vi "UtilityProcessCSVStringTo2DArray.vi"(8 "error in (no error)":errorcluster, 11 "CSV String":string) -> (0 "error out":errorcluster, 3 "Array":string[][](array[string]))   [LabVIEW 2019, in "flashcards.lvlib"]
uses:
  flashcards.lvlib
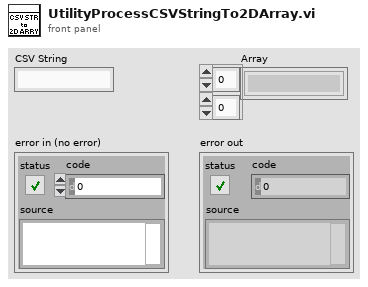
[diagram p1: front panel]
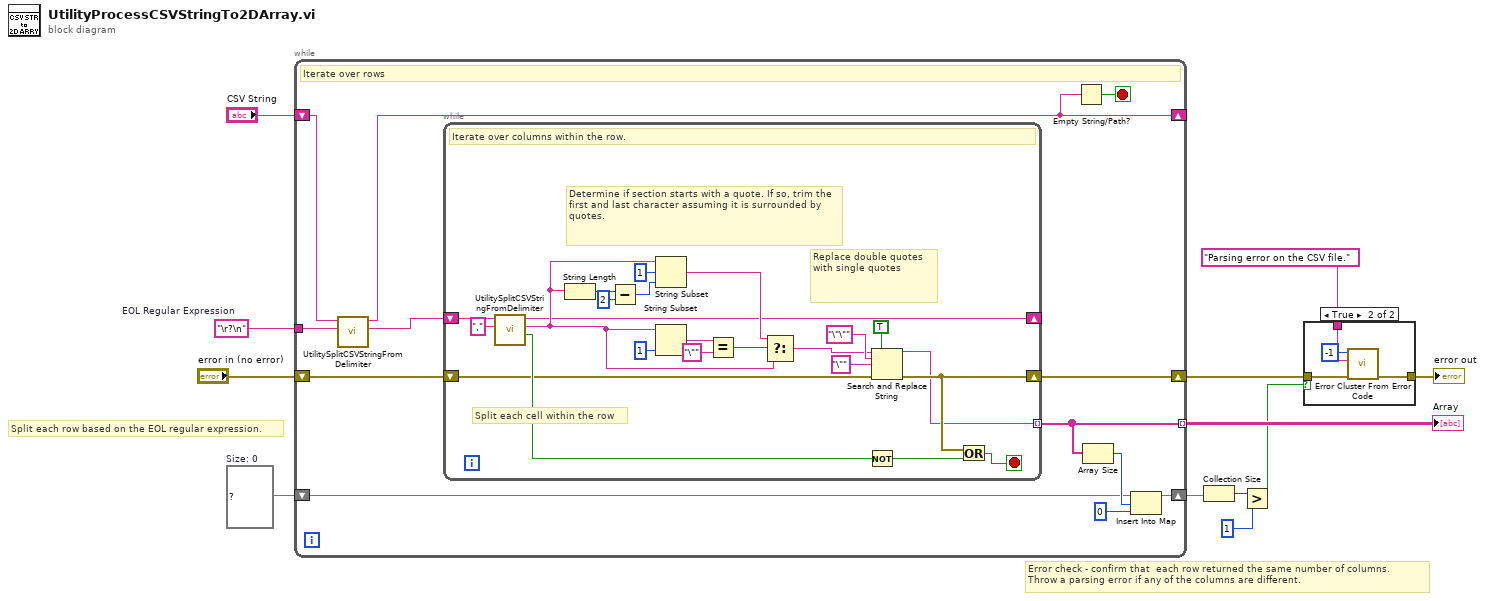
[diagram p0: block diagram]
diagram:
  w8 = map{i32, i32} {}  # Size: 0
  w12 = "\r?\n"  # EOL Regular Expression
  # "Error check - confirm that  each row returned the same number of columns.\nThrow a parsing error if any of the columns are different."
  # "Split each row based on the EOL regular expression."
  n1 = while {
    tunnel: w12 -> [w21]
    shift-right: [w23] -> w3
    shift-left: "error in (no error)" -> [w24]
    shift-right: [w20] -> _
    shift-left: "CSV String" -> [w19]
    tunnel: [w17] -> w11 mode=indexing
    shift-right: [w14] -> w7
    shift-left: w8 -> [w15]
    stop <- w22 stop-if-true
    # "Iterate over rows"
    n2 = call "UtilitySplitCSVStringFromDelimiter.vi"("Delimiter Regular Expression"=w21, "String in"=w19) -> ("Before Split"=w18:string, "After Split"=w20:string)  [unwired: 7 in, 1 out]
    n3 = while {
      shift-right: [w34] -> _
      shift-left: w18 -> [w33]
      shift-right: [w46] -> w23
      shift-left: w24 -> [w27]
      tunnel: [w25] -> w17 mode=indexing
      stop <- w47 stop-if-true
      # "Split each cell within the row"
      # "Determine if section starts with a quote. If so, trim the first and last character assuming it is surrounded by quotes."
      # "Replace double quotes with single quotes"
      # "Iterate over columns within the row."
      n4 = call "UtilitySplitCSVStringFromDelimiter.vi"("Delimiter Regular Expression"="," ("regular expression"), "String in"=w33) -> ("Match Found?"=w32:bool, "Before Split"=w35:string, "After Split"=w34:string)  [unwired: 7 in]
      n5 = String Length(string=w35) -> (length=w40:i32)
      n6 = Subtract(x=w40, y=2) -> (x-y=w38:i32)
      n7 = String Subset(string=w35, offset (0)=1, length (rest)=w38) -> (substring=w36:string)
      n8 = String Subset(string=w35, length (rest)=1 ("length (rest)")) -> (substring=w43:string)  [unwired: 1 in]
      n9 = Equal?(x=w43, y="\"") -> (x = y?=w41:bool)
      n10 = Select(t=w36, s=w41, f=w35) -> (s? t:f=w26:string)
      n11 = Not(x=w32) -> (.not. x?=w31:bool)
      n12 = Search and Replace String(replace all?=TRUE ("replace all? (F)"), input string=w26, search string="\"\"", replace string="\"" ("replace string (\"\")"), error in=w27) -> (result string=w25:string, error out=w46:errorcluster)  [unwired: 3 in, 2 out]
      n13 = Or(x=w46, y=w31) -> (x .or. y?=w47:bool)
    }
    n14 = Empty String/Path?(string/path=w20) -> (empty?=w22:bool)
    n15 = Array Size(array=w17) -> (size(s)=w16:i32)
    n16 = Insert Into Map(map in=w15, key=w16, value=0) -> (map out=w14:map{i32, i32})  [unwired: 2 out]
  }
  "Array" <- w11
  n17 = Collection Size(1:w7) -> (0:w6:i32)
  n18 = Greater?(x=w6, y=1) -> (0:w4:bool)
  n19 = case shown="True" w4 {
    tunnel: w3 -> [w48 w52]
    tunnel: [w48 w51] -> w2
    tunnel: "Parsing error on the CSV file." ("Append additional text (\"\")") -> [_ w50]
    frame False {
    }
    frame True {
      n20 = call <vilib>:"Error Cluster From Error Code.vi"("error in (no error)"=w52, "error message (\"\")"=w50, "error code (0)"=-1) -> ("error out"=w51:errorcluster)  [unwired: 6 in]
    }
  }
  "error out" <- w2
